vi "create.vi"(8 "error in (no error)":errorcluster, 10 "configuration":T1, 11 "json.provider in":refnum<class "json.provider.lvclass">) -> (0 "error out":errorcluster, 3 "json.provider out":refnum<class "json.provider.lvclass">)   [LabVIEW 2021, in "json.provider.lvclass"]
uses:
  json.provider.lvclass
  system.logging/configuration.ctl
  system.logging.provider.lvclass
  json.provider.lvclass/json.provider.ctl
  system.logging/system.logging.lvclass
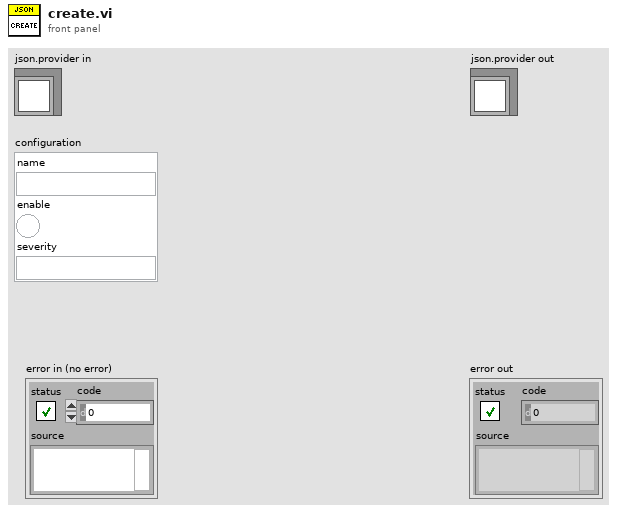
[diagram p1: front panel]
types:
  T1 = typedef "system.logging.lvclass/configuration.ctl" = cluster{"name":string, "enable":bool, "severity":string}
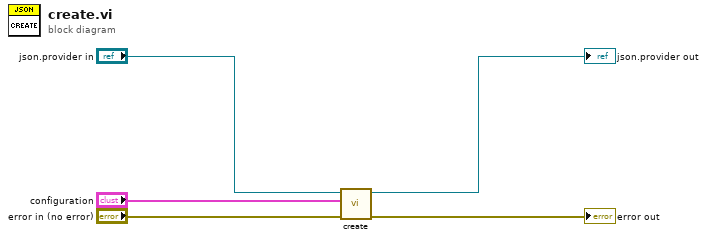
[diagram p0: block diagram]
diagram:
  n1 = call-parent "create.vi"("error in (no error)"="error in (no error)", "configuration"="configuration", "system.logging.provider in"="json.provider in") -> ("error out"=→"error out":errorcluster, "system.logging.provider out"=→"json.provider out":refnum<class "json.provider.lvclass">)  [unwired: 7 in]
